vi "PXI DAQ.vi"(1 "Action":T1, 7 "Cycles In":i32, 11 "error in (no error)":errorcluster) -> (8 "Buffers played":i32, 14 "method":T1, 15 "error out":errorcluster)   [LabVIEW 2020]
uses:
  Type Defs/PXI DAQ-Actions.ctl
  Type Defs/DAQ Write State enum.ctl
  Type Defs/Task Struct.ctl
  PXI Globals.vi
panel:
  out "#cycles":i32
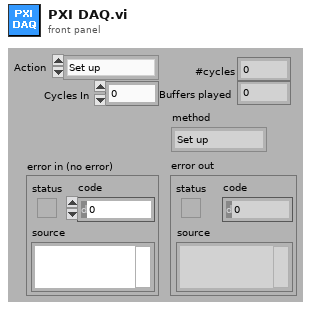
[diagram p1: front panel]
types:
  T1 = typedef "PXI DAQ-Actions.ctl" = enum16{"Set up", "Measure", "Trigger", "AO Queue", "Clean up"}
  T2 = typedef "DAQ Write State enum.ctl" = enum16{"Normal", "Ramp down", "Zero buffers", "Done"}
  T3 = typedef "Task Struct.ctl" = cluster{"Task name":string, "Task":refnum<k21>, "Dual-channel task?":bool, "Regenerate?":bool, "Clear?":bool}
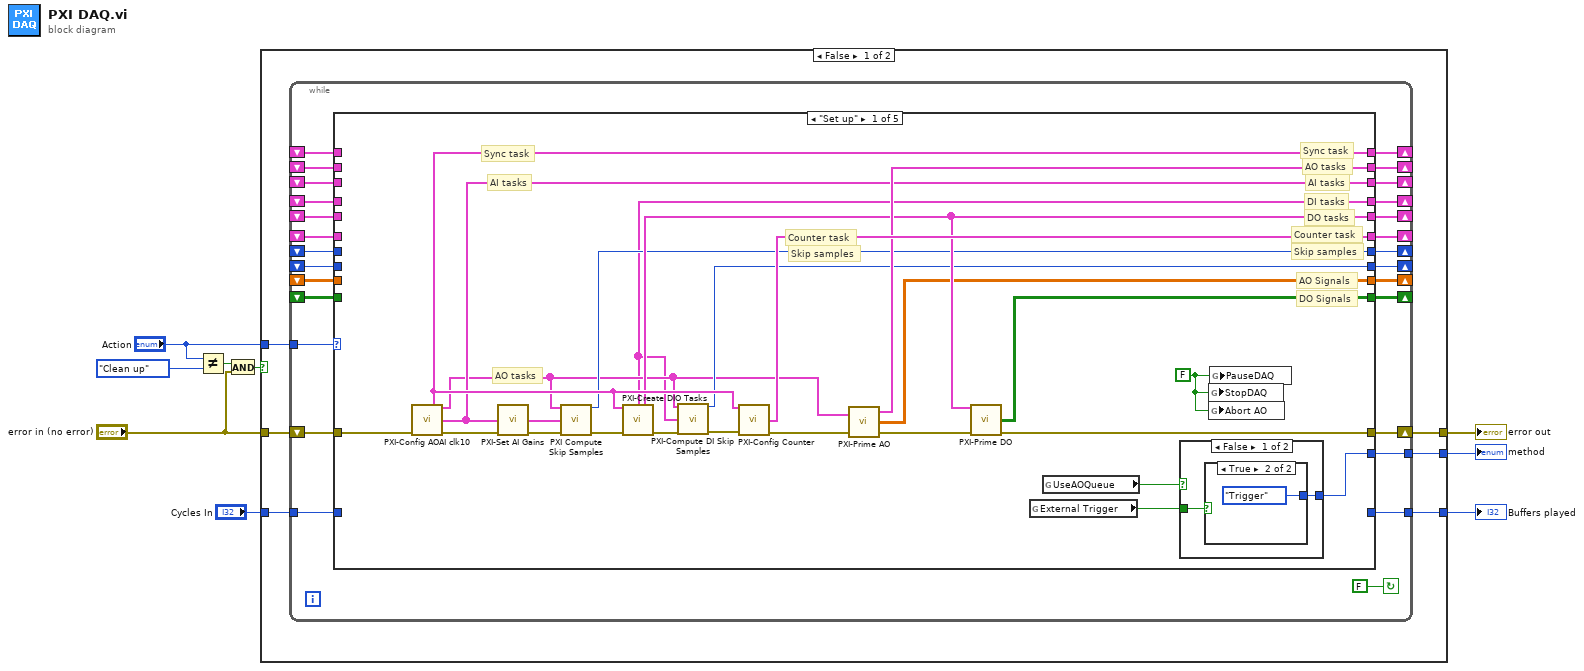
[diagram p0: block diagram]
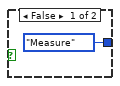
[diagram p2: hidden frame]
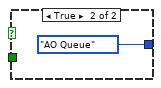
[diagram p3: hidden frame]
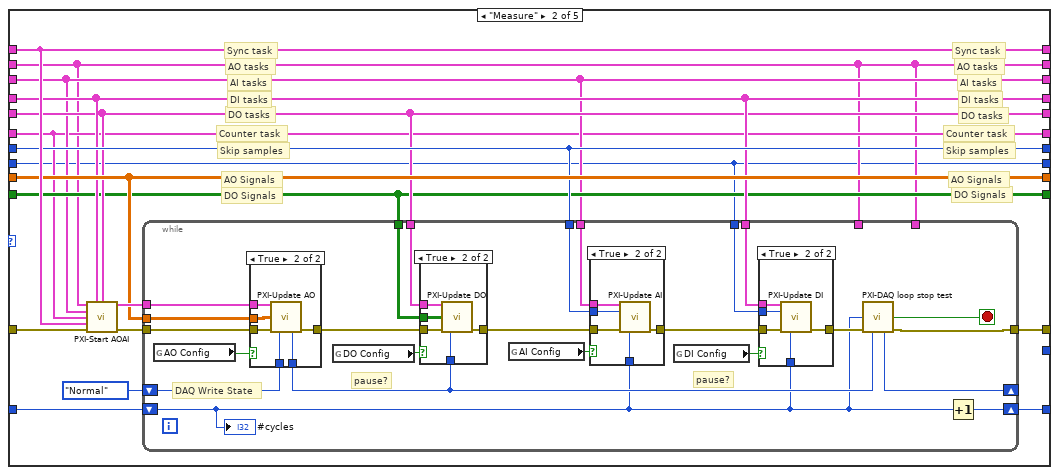
[diagram p4: hidden frame]
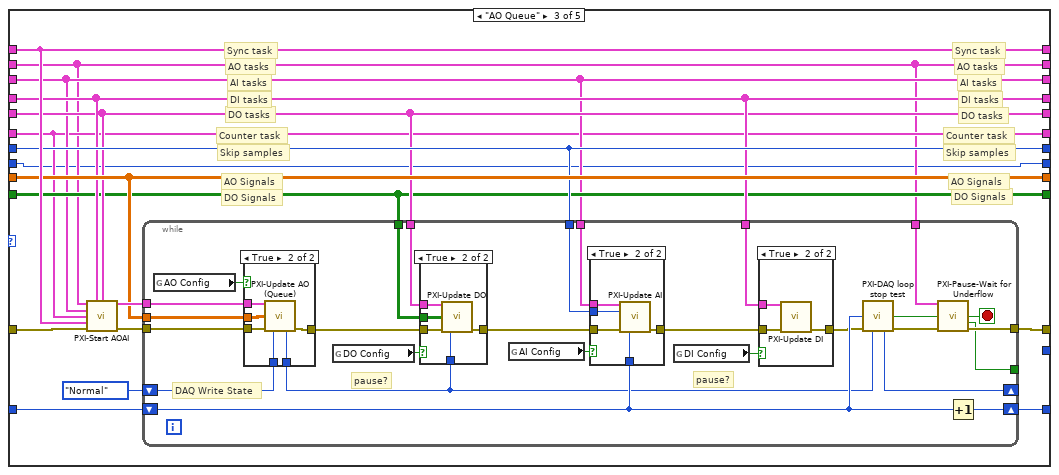
[diagram p9: hidden frame]
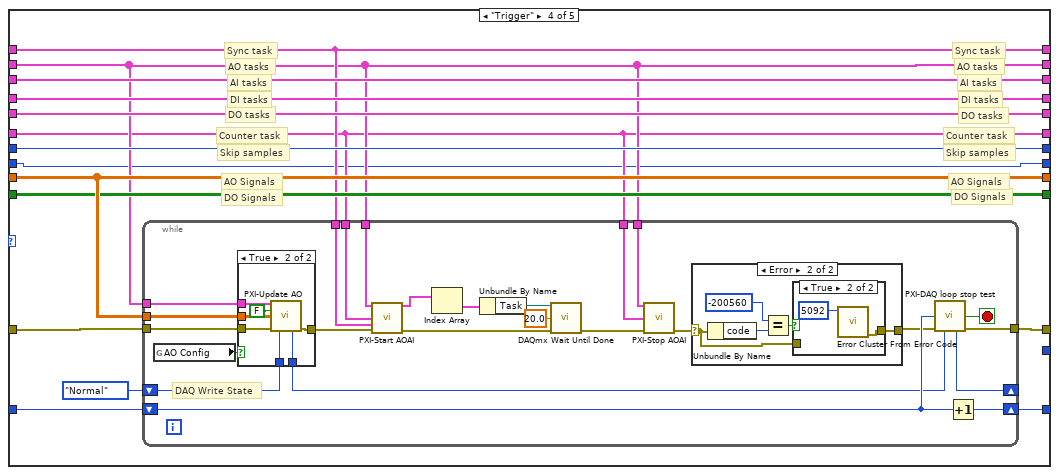
[diagram p14: hidden frame]
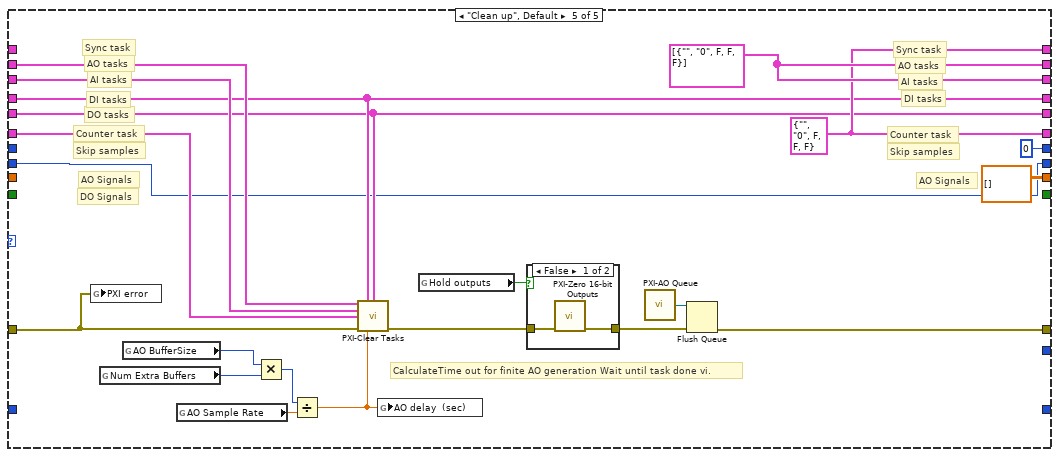
[diagram p18: hidden frame]
diagram:
  n1 = Not Equal?(x="Action", y=PXI_DAQ-Actions."Clean up") -> (x != y?=w8:bool)
  n2 = And(x=w8, y="error in (no error)") -> (x .and. y?=w7:bool)
  n3 = case shown="False" w7 {
    tunnel: "error in (no error)" -> [w15 w290]
    tunnel: [w14 w290] -> w6
    tunnel: "Action" -> [w13 _]
    tunnel: [w12 _] -> w5
    tunnel: "Cycles In" -> [w11 _]
    tunnel: [w10 _] -> w1
    frame False {
      n4 = while {
        shift-right: [w39] -> w14
        shift-left: w15 -> [w41]
        tunnel: w13 -> [w40]
        shift-right: [w38] -> _
        shift-left: _ -> [w35]
        shift-right: [w37] -> _
        shift-left: _ -> [w34]
        shift-right: [w36] -> _
        shift-left: _ -> [w33]
        shift-right: [w32] -> _
        shift-left: _ -> [w31]
        shift-right: [w30] -> _
        shift-left: _ -> [w29]
        shift-right: [w28] -> _
        shift-left: _ -> [w27]
        shift-right: [w26] -> _
        shift-left: _ -> [w25]
        shift-right: [w24] -> _
        shift-left: _ -> [w23]
        shift-right: [w22] -> _
        shift-left: _ -> [w21]
        tunnel: [w20] -> w12
        tunnel: w11 -> [w19]
        tunnel: [w18] -> w10
        shift-right: [w17] -> _
        shift-left: _ -> [w16]
        stop <- FALSE ("stop") continue-if-true
        n5 = case shown="\"Set up\"" w40 {
          tunnel: w41 -> [w64 w88 w155 w213 w271]
          tunnel: [w59 w85 w152 w222 w268] -> w39
          tunnel: [w62 w89 w156 w211 w284] -> w38
          tunnel: [w63 w74 w141 w210 w285] -> w37
          tunnel: [w58 w78 w145 w212 w285] -> w36
          tunnel: w35 -> [_ w89 w156 w211 _]
          tunnel: w34 -> [_ w74 w141 w210 w277]
          tunnel: w33 -> [_ w78 w145 w212 w276]
          tunnel: [w66 w75 w142 w209 w284] -> w32
          tunnel: w31 -> [_ w75 w142 w209 w275]
          tunnel: [w49 w82 w149 w219 0 ("MaxPresentations")] -> w30
          tunnel: w29 -> [_ w82 w149 w219 _]
          tunnel: [w50 w84 w151 w221 dbl[][] [] ("AO Waveforms")] -> w28
          tunnel: w27 -> [_ w84 w151 w221 _]
          tunnel: [w43 w81 w148 w218 w274] -> w26
          tunnel: w25 -> [_ w81 w148 w218 w274]
          tunnel: [w61 w80 w147 w217 w273] -> w24
          tunnel: w23 -> [_ w80 w147 w217 w273]
          tunnel: [w51 w79 w146 w216 _] -> w22
          tunnel: w21 -> [_ w79 w146 w216 _]
          tunnel: [_ w77 w144 w215 _] -> w20
          tunnel: w19 -> [_ w76 w143 w214 _]
          tunnel: [w53 _ _ _ _] -> w18
          tunnel: [w48 w73 w140 w208 w266] -> w17
          tunnel: w16 -> [_ w73 w140 w208 w266]
          frame "Set up" {
            w57 = FALSE ("Pause")
            # "DO Signals"
            # "DO tasks"
            # "DI tasks"
            # "AO tasks"
            # "AO Signals"
            # "Skip samples"
            # "Counter task"
            # "AI tasks"
            # "Sync task"
            # "Skip samples"
            # "Counter task"
            # "AI tasks"
            # "AO tasks"
            # "Sync task"
            n6 = call "PXI-Config AOAI clk10.vi"("error in (no error)"=w64) -> ("Sync Task"=w62:T3, "AO Tasks"=w44:T3[], "AI Tasks"=w58:T3[], "error out"=w65:errorcluster)  [unwired: 11 in]
            n7 = call "PXI-Set AI Gains.vi"("AI Tasks"=w58, "error in (no error)"=w65) -> ("AI Tasks out"=w55:T3[], "error out"=w56:errorcluster)  [unwired: 12 in]
            n8 = call "PXI Compute Skip Samples.vi"("AO Tasks"=w44, "AI Tasks"=w55, "error in (no error)"=w56) -> ("Skip Samples"=w49:i32, "error out"=w47:errorcluster)  [unwired: 11 in]
            n9 = call "PXI-Create DIO Tasks.vi"("Sync Task"=w62, "error in (no error)"=w47) -> ("DI Tasks"=w43:T3[], "DO Tasks"=w61:T3[], "error out"=w46:errorcluster)  [unwired: 11 in]
            n10 = call "PXI-Compute DI Skip Samples.vi"("AO Tasks"=w44, "DI Tasks"=w43, "error in (no error)"=w46) -> ("Skip Samples"=w48:i32, "error out"=w45:errorcluster)  [unwired: 11 in]
            n11 = call "PXI-Config Counter.vi"("Sync Task"=w62, "error in (no error)"=w45) -> ("Counter Task"=w66:T3, "error out"=w67:errorcluster)  [unwired: 12 in]
            n12 = call "PXI-Prime AO.vi"("AO Tasks"=w44, "error in"=w67) -> ("AO Tasks out"=w63:T3[], "AO Waveforms"=w50:dbl[][], "error out"=w60:errorcluster)
            n13 = call "PXI-Prime DO.vi"("DO Tasks"=w61, "error in"=w60) -> ("DO Waveforms"=w51:bool[][], "error out"=w59:errorcluster)  [unwired: 11 in, 1 out]
            n14 = global read "PXI Globals.vi" "External Trigger"() -> (w52:bool)
            n15 = global read "PXI Globals.vi" "UseAOQueue"() -> (w54:bool)
            n16 = case shown="False" w54 {
              tunnel: [w68 PXI_DAQ-Actions."AO Queue" ("Action")] -> w53
              tunnel: w52 -> [w69 _]
              frame False {
                n17 = case shown="True" w69 {
                  tunnel: [PXI_DAQ-Actions."Measure" ("Action") PXI_DAQ-Actions."Trigger" ("Action")] -> w68
                  frame False {
                  }
                  frame True {
                  }
                }
              }
              frame True {
              }
            }
            n18 = global write "PXI Globals.vi" "StopDAQ"(w57) -> ()
            n19 = global write "PXI Globals.vi" "Abort AO"(w57) -> ()
            n20 = global write "PXI Globals.vi" "PauseDAQ"(w57) -> ()
          }
          frame "Measure" {
            # "DO Signals"
            # "DO Signals"
            # "DO tasks"
            # "DO tasks"
            # "DI tasks"
            # "DI tasks"
            # "AO Signals"
            # "Skip samples"
            # "Counter task"
            # "AI tasks"
            # "Sync task"
            # "AO tasks"
            # "AO Signals"
            # "Skip samples"
            # "Counter task"
            # "AI tasks"
            # "Sync task"
            # "AO tasks"
            n21 = call "PXI-Start AOAI.vi"("AO Tasks"=w74, "DI Tasks"=w81, "DO Tasks"=w80, "AI Tasks"=w78, "Counter Task"=w75, "Sync Task"=w89, "error in (no error)"=w88) -> ("AO Tasks out"=w86:T3[], "error out"=w87:errorcluster)  [unwired: 7 in]
            n22 = while {
              tunnel: w86 -> [w112]
              tunnel: w84 -> [w113]
              tunnel: w78 -> [w111]
              tunnel: w82 -> [w110]
              shift-right: [w108] -> _
              shift-left: DAQ_Write_State_enum."Normal" ("DAQ Write State") -> [w94]
              tunnel: w81 -> [w104]
              tunnel: w80 -> [w101]
              tunnel: w79 -> [w100]
              tunnel: w87 -> [w92]
              tunnel: [w99] -> w85
              tunnel: w74 -> [_]
              shift-right: [w97] -> w77
              shift-left: w76 -> [w90]
              tunnel: w74 -> [_]
              tunnel: w73 -> [w91]
              stop <- w98 stop-if-true
              # "pause?"
              # "pause?"
              # "DAQ Write State"
              n23 = global read "PXI Globals.vi" "AO Config"() -> (w109:bool)
              n24 = case shown="True" w109 {
                tunnel: w113 -> [_ w139]
                tunnel: w112 -> [_ w138]
                tunnel: [w132 w137] -> w96
                tunnel: w94 -> [w133 w136]
                tunnel: [w133 w135] -> w93
                tunnel: w92 -> [w132 w134]
                frame False {
                }
                frame True {
                  n25 = call "PXI-Update AO.vi"("AO Tasks"=w138, "AO Waveforms"=w139, "error in (no error)"=w134, "DAQ Write State"=w136) -> ("DAQ Write State Out"=w135:T2, "error out"=w137:errorcluster)  [unwired: 9 in, 1 out]
                }
              }
              n26 = global read "PXI Globals.vi" "DO Config"() -> (w103:bool)
              n27 = case shown="True" w103 {
                tunnel: w96 -> [w114 w119]
                tunnel: [w114 w118] -> w102
                tunnel: w93 -> [_ w117]
                tunnel: w101 -> [_ w116]
                tunnel: w100 -> [_ w115]
                frame False {
                }
                frame True {
                  n28 = call "PXI-Update DO.vi"("DO Tasks"=w116, "DO Waveforms"=w115, "error in (no error)"=w119, "DAQ Write State"=w117) -> ("error out"=w118:errorcluster)  [unwired: 11 in]
                }
              }
              n29 = global read "PXI Globals.vi" "AI Config"() -> (w107:bool)
              n30 = case shown="True" w107 {
                tunnel: w102 -> [w126 w131]
                tunnel: [w126 w130] -> w105
                tunnel: w111 -> [_ w129]
                tunnel: w110 -> [_ w128]
                tunnel: w90 -> [_ w127]
                frame False {
                }
                frame True {
                  n31 = call "PXI-Update AI.vi"("AI Tasks"=w129, "Skip samples"=w128, "error in (no error)"=w131, "cycle"=w127) -> ("error out"=w130:errorcluster)  [unwired: 11 in]
                }
              }
              n32 = global read "PXI Globals.vi" "DI Config"() -> (w106:bool)
              n33 = case shown="True" w106 {
                tunnel: w105 -> [w120 w125]
                tunnel: [w120 w124] -> w95
                tunnel: w104 -> [_ w123]
                tunnel: w91 -> [_ w122]
                tunnel: w90 -> [_ w121]
                frame False {
                }
                frame True {
                  n34 = call "PXI-Update DI.vi"("DI Tasks"=w123, "Skip samples"=w122, "error in (no error)"=w125, "cycle"=w121) -> ("error out"=w124:errorcluster)  [unwired: 11 in]
                }
              }
              n35 = call "PXI-DAQ loop stop test.vi"("Cycle"=w90, "error in (no error)"=w95, "DAQ Write State"=w93) -> ("Stop?"=w98:bool, "DAQ Write State out"=w108:T2, "error out"=w99:errorcluster)  [unwired: 10 in]
              n36 = Increment(x=w90) -> (x+1=w97:i32)
              "#cycles" <- w90
            }
          }
          frame "AO Queue" {
            # "DO Signals"
            # "DO Signals"
            # "DO tasks"
            # "DO tasks"
            # "DI tasks"
            # "DI tasks"
            # "AO Signals"
            # "Skip samples"
            # "Counter task"
            # "AI tasks"
            # "Sync task"
            # "AO tasks"
            # "AO Signals"
            # "Skip samples"
            # "Counter task"
            # "AI tasks"
            # "Sync task"
            # "AO tasks"
            n37 = call "PXI-Start AOAI.vi"("AO Tasks"=w141, "DI Tasks"=w148, "DO Tasks"=w147, "AI Tasks"=w145, "Counter Task"=w142, "Sync Task"=w156, "error in (no error)"=w155) -> ("AO Tasks out"=w153:T3[], "error out"=w154:errorcluster)  [unwired: 7 in]
            n38 = while {
              tunnel: w153 -> [w182]
              tunnel: w151 -> [w183]
              tunnel: w145 -> [w181]
              tunnel: w149 -> [w180]
              shift-right: [w178] -> _
              shift-left: DAQ_Write_State_enum."Normal" ("DAQ Write State") -> [w159]
              tunnel: w148 -> [w174]
              tunnel: w147 -> [w171]
              tunnel: w146 -> [w170]
              tunnel: w154 -> [w157]
              tunnel: [w167] -> w152
              tunnel: w141 -> [w165]
              tunnel: [w164] -> _
              shift-right: [w162] -> w144
              shift-left: w143 -> [w163]
              stop <- w169 stop-if-true
              # "pause?"
              # "pause?"
              # "DAQ Write State"
              n39 = global read "PXI Globals.vi" "AO Config"() -> (w179:bool)
              n40 = case shown="True" w179 {
                tunnel: w183 -> [_ w207]
                tunnel: w182 -> [_ w206]
                tunnel: [w200 w205] -> w161
                tunnel: w159 -> [w201 w204]
                tunnel: [w201 w203] -> w158
                tunnel: w157 -> [w200 w202]
                frame False {
                }
                frame True {
                  n41 = call "PXI-Update AO (Queue).vi"("AO Tasks"=w206, "AO Waveforms"=w207, "error in (no error)"=w202, "DAQ Write State"=w204) -> ("DAQ Write State Out"=w203:T2, "error out"=w205:errorcluster)  [unwired: 10 in]
                }
              }
              n42 = global read "PXI Globals.vi" "DO Config"() -> (w173:bool)
              n43 = case shown="True" w173 {
                tunnel: w161 -> [w184 w189]
                tunnel: [w184 w188] -> w172
                tunnel: w158 -> [_ w187]
                tunnel: w171 -> [_ w186]
                tunnel: w170 -> [_ w185]
                frame False {
                }
                frame True {
                  n44 = call "PXI-Update DO.vi"("DO Tasks"=w186, "DO Waveforms"=w185, "error in (no error)"=w189, "DAQ Write State"=w187) -> ("error out"=w188:errorcluster)  [unwired: 11 in]
                }
              }
              n45 = global read "PXI Globals.vi" "AI Config"() -> (w177:bool)
              n46 = case shown="True" w177 {
                tunnel: w172 -> [w194 w199]
                tunnel: [w194 w198] -> w175
                tunnel: w181 -> [_ w197]
                tunnel: w180 -> [_ w196]
                tunnel: w163 -> [_ w195]
                frame False {
                }
                frame True {
                  n47 = call "PXI-Update AI.vi"("AI Tasks"=w197, "Skip samples"=w196, "error in (no error)"=w199, "cycle"=w195) -> ("error out"=w198:errorcluster)  [unwired: 11 in]
                }
              }
              n48 = global read "PXI Globals.vi" "DI Config"() -> (w176:bool)
              n49 = case shown="True" w176 {
                tunnel: w175 -> [w190 w193]
                tunnel: [w190 w192] -> w160
                tunnel: w174 -> [_ w191]
                frame False {
                }
                frame True {
                  n50 = call "PXI-Update DI.vi"("DI Tasks"=w191, "error in (no error)"=w193) -> ("error out"=w192:errorcluster)  [unwired: 13 in]
                }
              }
              n51 = call "PXI-DAQ loop stop test.vi"("Cycle"=w163, "error in (no error)"=w160, "DAQ Write State"=w158) -> ("Stop?"=w166:bool, "DAQ Write State out"=w178:T2, "error out"=w168:errorcluster)  [unwired: 10 in]
              n52 = call "PXI-Pause-Wait for Underflow.vi"("AO Tasks"=w165, "Abort?"=w166, "error in (no error)"=w168) -> ("Abort out"=w169:bool, "Pause out"=w164:bool, "error out"=w167:errorcluster)  [unwired: 10 in]
              n53 = Increment(x=w163) -> (x+1=w162:i32)
            }
          }
          frame "Trigger" {
            # "DO Signals"
            # "DO Signals"
            # "DO tasks"
            # "DO tasks"
            # "DI tasks"
            # "DI tasks"
            # "AO Signals"
            # "Skip samples"
            # "Counter task"
            # "AI tasks"
            # "Sync task"
            # "AO tasks"
            # "AO Signals"
            # "Skip samples"
            # "Counter task"
            # "AI tasks"
            # "Sync task"
            # "AO tasks"
            n54 = while {
              tunnel: w210 -> [w246]
              tunnel: w221 -> [w247]
              shift-right: [w244] -> _
              shift-left: DAQ_Write_State_enum."Normal" ("DAQ Write State") -> [w241]
              tunnel: w213 -> [w239]
              tunnel: [w238] -> w222
              shift-right: [w242] -> w215
              shift-left: w214 -> [w243]
              tunnel: w210 -> [w235]
              tunnel: w211 -> [w234]
              tunnel: w209 -> [w229]
              tunnel: w210 -> [w228]
              tunnel: w209 -> [w227]
              stop <- w237 stop-if-true
              # "DAQ Write State"
              n55 = global read "PXI Globals.vi" "AO Config"() -> (w245:bool)
              n56 = case shown="True" w245 {
                tunnel: w247 -> [_ w265]
                tunnel: w246 -> [_ w264]
                tunnel: [w257 w263] -> w236
                tunnel: w241 -> [w258 w262]
                tunnel: [w258 w261] -> w240
                tunnel: w239 -> [w257 w260]
                frame False {
                }
                frame True {
                  n57 = call "PXI-Update AO.vi"("AO Tasks"=w264, "Wait for Buffer Space (T)?"=FALSE, "AO Waveforms"=w265, "error in (no error)"=w260, "DAQ Write State"=w262) -> ("DAQ Write State Out"=w261:T2, "error out"=w263:errorcluster)  [unwired: 8 in, 1 out]
                }
              }
              n58 = call "PXI-Start AOAI.vi"("AO Tasks"=w235, "Counter Task"=w229, "Sync Task"=w234, "error in (no error)"=w236) -> ("AO Tasks out"=w233:T3[], "error out"=w225:errorcluster)  [unwired: 10 in]
              n59 = Index Array(array=w233) -> (element=w232:T3)  [unwired: 1 in]
              n60 = Unbundle By Name(w232) -> ("Task"=w231:refnum<k21>)
              n61 = call <vilib>:"DAQmx Wait Until Done.vi"("task/channels in"=w231, "timeout (sec)"=20.0, "error in"=w225) -> ("error out"=w226:errorcluster)  [unwired: 11 in, 1 out]
              n62 = call "PXI-Stop AOAI.vi"("AO Tasks"=w228, "Counter Task"=w227, "error in (no error)"=w226) -> ("error out"=w224:errorcluster)  [unwired: 12 in]
              n63 = case shown="Error" w224 {
                selector: w224 -> [w248 w249]
                tunnel: [w248 w250] -> w223
                frame No Error {
                }
                frame Error {
                  n64 = Unbundle By Name(w249) -> ("code"=w253:i32)
                  n65 = Equal?(x=-200560, y=w253) -> (x = y?=w251:bool)
                  n66 = case shown="True" w251 {
                    tunnel: [w254 w256] -> w250
                    tunnel: w249 -> [w254 _]
                    frame False {
                    }
                    frame True {
                      n67 = call <vilib>:"Error Cluster From Error Code.vi"("error code (0)"=5092) -> ("error out"=w256:errorcluster)  [unwired: 8 in]
                    }
                  }
                }
              }
              n68 = call "PXI-DAQ loop stop test.vi"("Cycle"=w243, "error in (no error)"=w223, "DAQ Write State"=w240) -> ("Stop?"=w237:bool, "DAQ Write State out"=w244:T2, "error out"=w238:errorcluster)  [unwired: 10 in]
              n69 = Increment(x=w243) -> (x+1=w242:i32)
            }
          }
          frame "Clean up", Default {
            w285 = T3[] [{"Task name"="", "Task"="0", "Dual-channel task?"=FALSE, "Regenerate?"=FALSE, "Clear?"=FALSE}] ("AO Tasks")
            w284 = T3 {"Task name"="", "Task"="0", "Dual-channel task?"=FALSE, "Regenerate?"=FALSE, "Clear?"=FALSE} ("Sync Task")
            # "DO Signals"
            # "DO tasks"
            # "DI tasks"
            # "DI tasks"
            # "AO Signals"
            # "Skip samples"
            # "Counter task"
            # "AI tasks"
            # "Sync task"
            # "AO tasks"
            # "AO Signals"
            # "Skip samples"
            # "Counter task"
            # "AI tasks"
            # "Sync task"
            # "AO tasks"
            # "CalculateTime out for finite AO generation Wait until task done vi."
            n70 = global write "PXI Globals.vi" "PXI error"(w271) -> ()
            n71 = global read "PXI Globals.vi" "Num Extra Buffers"() -> (w280:i32)
            n72 = global read "PXI Globals.vi" "AO BufferSize"() -> (w281:i32)
            n73 = global read "PXI Globals.vi" "AO Sample Rate"() -> (w279:dbl)
            n74 = Multiply(x=w281, y=w280) -> (x*y=w282:i32)
            n75 = Divide(x=w282, y=w279) -> (x/y=w278:dbl)
            n76 = call "PXI-Clear Tasks.vi"("AO Tasks"=w277, "DI Tasks"=w274, "DO Tasks"=w273, "AI Tasks"=w276, "Counter Task"=w275, "error in (no error)"=w271, "timeout (sec)"=w278) -> ("error out"=w272:errorcluster)  [unwired: 8 in]
            n77 = global write "PXI Globals.vi" "AO delay  (sec)"(w278) -> ()
            n78 = global read "PXI Globals.vi" "Hold outputs"() -> (w267:bool)
            n79 = case shown="False" w267 {
              tunnel: w272 -> [w288 w289]
              tunnel: [w287 w289] -> w270
              frame False {
                n80 = call "PXI-Zero 16-bit Outputs.vi"("error in (no error)"=w288) -> ("error out"=w287:errorcluster)  [unwired: 10 in]
              }
              frame True {
              }
            }
            n81 = call "PXI-AO Queue.vi"() -> ("Queue"=w269:refnum<queue>)  [unwired: 15 in]
            n82 = Flush Queue(queue=w269, error in (no error)=w270) -> (error out=w268:errorcluster)  [unwired: 2 out]
          }
        }
      }
    }
    frame True {
    }
  }
  "error out" <- w6
  "Buffers played" <- w5
  "method" <- w1
